vi "Derivative of intensity graph V1.0.vi"() -> ()   [LabVIEW 2016]
uses:
  <vilib>/Utility/miscctls.llb/LVOffsetAndMultiplierTypeDef.ctl
  <vilib>/Analysis/NI_AALPro.lvlib
panel:
  in  "Cursor.Visible ? 2":bool
  in  "Cursor.Visible ?":bool
  in  "Tab Control":T1(tab)=enum."Index linecut curve"
  out "All derivatives":cluster{dbl[], dbl[]}[](graph)
  out "All Data":cluster{dbl[], dbl[]}[](graph)
  out "Linecut of Data":dbl[](graph)=[-5.165548349618656e-08, -5.159647504832888e-08, -5.1548035526661304e-08, -5.148192440940621e-08, -5.1383318345099665e-08, -5.1286353274798515e-08, -5.1218371208053366e-08, -5.116268641366293e-08, -5.109130548013824e-08, -5.098742924360193e-08, -5.085517949337487e-08, -5.074484750756666e-08, -5.068211876052946e-08, -5.0617670460310636e-08, -5.052406640959861e-08, -5.0408820269667306e-08, -5.0295145102842986e-08, -5.022248512748516e-08, -5.0180627286568036e-08, -5.0122652084791704e-08, -5.0040971452737534e-08, -4.995074993072835e-08, -4.985441092029686e-08, -4.9765018529941685e-08, -4.9675366699941365e-08, -4.9564350089994913e-08, -4.947029200628265e-08, -4.941443648162086e-08, -4.9353383054520915e-08, -4.926843157132916e-08, -4.9167242647363985e-08, -4.9065280874750254e-08, -4.899516497811031e-08, -4.8946122255576085e-08, -4.8863182385243175e-08, -4.87432636505986e-08, -4.862626638254201e-08, -4.853802567987668e-08, -4.848543315041591e-08, -4.8426769491768916e-08, -4.8331422602193806e-08, -4.823856670019399e-08, -4.816860860479887e-08, -4.8102166770697064e-08, -4.802987848539934e-08, -4.793796883789405e-08, -4.781875406953681e-08, -4.771223992954938e-08, -4.763483877438248e-08, -4.754388789459166e-08, -4.7432043547268955e-08, -4.731969281618781e-08, -4.722403394999117e-08, -4.7168647720075765e-08, -4.7134074086052784e-08, -4.707674724162832e-08, -4.699229851817311e-08, -4.689341985858352e-08, -4.6792670550280276e-08, -4.670473526864287e-08, -4.661186261528778e-08, -4.6503181017626753e-08, -4.641773033998275e-08, -4.636383873714532e-08, -4.6302239747671046e-08, -4.6219178803954826e-08, -4.611830349088384e-08, -4.6008475468028e-08, -4.591595258925939e-08, -4.584258830545454e-08, -4.57565406467377e-08, -4.565177461639157e-08, -4.55465010012447e-08, -4.544778298049394e-08, -4.537022560498973e-08, -4.5294561734900574e-08, -4.51842662663245e-08, -4.50710244054238e-08, -4.498678438032247e-08, -4.4916903048519334e-08, -4.483955437949311e-08, -4.474237791949989e-08, -4.464581168364172e-08, -4.4578839630322026e-08, -4.453545408463023e-08, -4.449345444981521e-08, -4.4445241282709766e-08, -4.4385705029112496e-08, -4.432274008638454e-08, -4.428047295002768e-08, -4.4231581361464624e-08, -4.413781408332821e-08, -4.402319403819412e-08, -4.392601686965633e-08, -4.385863063612994e-08, -4.3801470329639925e-08, -4.371464154197799e-08, -4.3585122865865986e-08, -4.3460048915201843e-08, -4.337618346856069e-08, -4.331416381624075e-08, -4.3252734547339044e-08, -4.3178842629403106e-08, -4.309602498723277e-08, -4.302060377664933e-08, -4.2945197911975524e-08, -4.2853584205840277e-08, -4.274446242764889e-08, -4.2631638334099326e-08, -4.253330374780791e-08, -4.2464012166724194e-08, -4.240684288478342e-08, -4.2325780772523794e-08, -4.222915038694011e-08, -4.2144893670544885e-08, -4.207001139198109e-08, -4.197951570204532e-08, -4.186293064936822e-08, -4.175155954277796e-08, -4.167633885796429e-08, -4.161761529242304e-08, -4.154372126835706e-08, -4.145120843461285e-08, -4.134665858173513e-08, -4.1249818939228537e-08, -4.11753684692289e-08, -4.1091024655823804e-08, -4.0975882847820176e-08, -4.085292266614936e-08, -4.0742754209786083e-08, -4.0659009748824605e-08, -4.0591286871812844e-08, -4.050720526388395e-08, -4.040783116052655e-08, -4.032631292398029e-08, -4.026575037929934e-08, -4.020033236599087e-08, -4.0118832371796704e-08, -4.0017884803601105e-08, -3.992062274168703e-08, -3.985915456501376e-08, -3.980910502914425e-08, -3.973949905215017e-08, -3.965749923353381e-08, -3.9573475035086906e-08, -3.949800011829344e-08, -3.942955342618568e-08, -3.933789965676449e-08, -3.922077992498132e-08, -3.912218722513151e-08, -3.905296257274388e-08, -3.8992130231414786e-08, -3.892327433845437e-08, -3.882445359006842e-08, -3.871234332414376e-08, -3.861881128126975e-08, -3.853639914523126e-08, -3.8456071626752795e-08, -3.837040236955144e-08, -3.827509069359456e-08, -3.820089270678577e-08, -3.815510009217847e-08, -3.8094101565054805e-08, -3.8009604245617294e-08, -3.791565039339955e-08, -3.781772114946437e-08, -3.7735527934768004e-08, -3.764922395007989e-08, -3.752862986218264e-08, -3.739858140578617e-08, -3.729352807309609e-08, -3.722253575841222e-08, -3.717238799522547e-08, -3.710583846146186e-08, -3.6999146668920645e-08, -3.6896083204113855e-08, -3.682999300151662e-08, -3.6769350479570105e-08, -3.669548253247852e-08, -3.660576874233244e-08, -3.6510217859818705e-08, -3.644074722814453e-08, -3.638687764944132e-08, -3.63104746678855e-08, -3.622213670971757e-08, -3.614929360125362e-08, -3.608616338943413e-08, -3.6024629858553956e-08, -3.594304806568941e-08, -3.5824548620609036e-08, -3.571563766462648e-08, -3.5646256883374475e-08, -3.558942283879134e-08, -3.5529346267070896e-08, -3.546135688902753e-08, -3.538546477475565e-08, -3.5322051576189394e-08, -3.5267963006398924e-08, -3.518638711023153e-08, -3.5077382944481216e-08, -3.496386175795827e-08, -3.485415433070339e-08, -3.4764224144210785e-08, -3.4679024766190425e-08, -3.4569988051248505e-08, -3.445874551980504e-08, -3.437124888411822e-08, -3.4303495045724726e-08, -3.4241346286418414e-08, -3.415948871180689e-08, -3.404952931528982e-08, -3.395058866948328e-08, -3.387865260122285e-08, -3.379725534723817e-08, -3.3704385993142976e-08, -3.3611839290837744e-08, -3.3515668636009095e-08, -3.344473917229437e-08, -3.3391339751836916e-08, -3.3305173758579915e-08, -3.319985030525287e-08, -3.311949351003222e-08, -3.305718996268877e-08, -3.299190902530916e-08, -3.29144757103662e-08, -3.281945470454397e-08, -3.2734986427922816e-08, -3.267696636548646e-08, -3.261974075041499e-08, -3.253445721133879e-08, -3.2405981533870483e-08, -3.226814349082853e-08, -3.216969703090513e-08, -3.210322902432682e-08, -3.2034629006142696e-08, -3.196009883122792e-08, -3.190026803540523e-08, -3.186337349867941e-08, -3.183599113260375e-08, -3.178096045409717e-08, -3.167867261642787e-08, -3.155730568256794e-08, -3.144426242929421e-08, -3.134959422836359e-08, -3.126876064771173e-08, -3.118366897239564e-08, -3.109381626446461e-08, -3.102917302092374e-08, -3.0995226421904973e-08, -3.095257095643533e-08, -3.087830071872433e-08, -3.077292081721096e-08, -3.0663717622016714e-08, -3.0586800674701934e-08, -3.0519909704341385e-08, -3.0428417060716443e-08, -3.031994915876719e-08, -3.021478359451866e-08, -3.012696058420965e-08, -3.005164622346892e-08, -2.99653646597268e-08, -2.98668895432762e-08, -2.9783009507890182e-08, -2.971327345593366e-08, -2.9638758475141435e-08, -2.955588599747759e-08, -2.946114270188039e-08, -2.9371640281182034e-08, -2.9303969115742402e-08, -2.9228801497056452e-08, -2.9123987631820767e-08, -2.9006876333603397e-08, -2.889923136094302e-08, -2.8816560698415582e-08, -2.8755997304679404e-08, -2.868170895711246e-08, -2.8578856589791276e-08, -2.8481290945567485e-08, -2.8404508937544794e-08, -2.8333305132237064e-08, -2.8251321719996546e-08, -2.814739759659086e-08, -2.804734616398572e-08, -2.7985450603452592e-08, -2.794437289599192e-08, -2.7880983143687256e-08, -2.778577975169189e-08, -2.7681281818291328e-08, -2.7601390761100666e-08, -2.756031474905914e-08, -2.7516809263284313e-08, -2.7445445010736174e-08, -2.736270737442078e-08, -2.727763117497891e-08, -2.7197946311589063e-08, -2.7120970747323493e-08, -2.702555948420715e-08, -2.6911600850550554e-08, -2.6816481307868774e-08, -2.6753150958716478e-08, -2.6693381712429233e-08, -2.660865438773106e-08, -2.6487032872792765e-08, -2.6365426120953676e-08, -2.627675831719376e-08, -2.6195161209717578e-08, -2.6099676084656567e-08, -2.5986396512281783e-08, -2.586723331071279e-08, -2.57835600655147e-08, -2.5738347234919e-08, -2.5679780414312992e-08, -2.559371639968789e-08, -2.5508309281632726e-08, -2.542956210418315e-08, -2.536115018323055e-08, -2.529184664632403e-08, -2.5195566825791836e-08, -2.5098662406207293e-08, -2.502554277389618e-08, -2.495268948619173e-08, -2.486601204395687e-08, -2.4760906463117536e-08, -2.464420797588273e-08, -2.455796873847971e-08, -2.4512213051135366e-08, -2.446195521773658e-08, -2.439636233437496e-08, -2.433152093401889e-08, -2.4266100296247668e-08, -2.4206929169608104e-08, -2.4136895052437086e-08, -2.4023778821815217e-08, -2.389002406014159e-08, -2.3774983953668427e-08, -2.368055336512477e-08, -2.3594935263044867e-08, -2.3503552165209706e-08, -2.3400009391694284e-08, -2.3319671183307225e-08, -2.326801413303854e-08, -2.3193851922599745e-08, -2.3089762124699337e-08, -2.2977748645147562e-08, -2.287448718729575e-08, -2.2805841155513513e-08, -2.275507350669239e-08, -2.267630666531651e-08, -2.2570712541859644e-08, -2.246884853943456e-08, -2.238319963142675e-08, -2.2312650014034985e-08, -2.2236937256527653e-08, -2.2136623645915668e-08, -2.203940093476987e-08, -2.1966393859608153e-08, -2.1896426138264626e-08, -2.18147422517242e-08, -2.1713288461790726e-08, -2.159774261507225e-08, -2.1505223158569168e-08, -2.1440090810716427e-08, -2.135722698071537e-08, -2.1250197110569697e-08, -2.1149508545896832e-08, -2.1069737284153304e-08, -2.1021898347111185e-08, -2.0981827622678454e-08, -2.0906481810483677e-08, -2.081466042512085e-08, -2.0744894567369e-08, -2.0697507729396806e-08, -2.0649843890112284e-08, -2.05641959407945e-08, -2.0432780646470743e-08, -2.0313373023767253e-08, -2.02326793255826e-08, -2.0150153361860347e-08, -2.0050066917813527e-08, -1.9938173404966368e-08, -1.9826619698408437e-08, -1.9741389771251036e-08, -1.967331644749085e-08, -1.95967010561806e-08, -1.9509851465096232e-08, -1.9424175649438275e-08, -1.9349724040100852e-08, -1.928195903350066e-08, -1.9198926357104354e-08, -1.909415070580926e-08, -1.900076819853445e-08, -1.8935772355636684e-08, -1.887772440051576e-08, -1.880849990199008e-08, -1.8716035876576055e-08, -1.8615119560084032e-08, -1.8539278487844478e-08, -1.8483419365321094e-08, -1.8415566535526765e-08, -1.832510175957605e-08, -1.8229381708746358e-08, -1.815210665530519e-08, -1.809714875140782e-08, -1.8025438038450318e-08, -1.7912436087299903e-08, -1.778786376701964e-08, -1.7676558631855445e-08, -1.758833435530881e-08, -1.751481606287522e-08, -1.7430530511459936e-08, -1.734447890831483e-08, -1.728565292959516e-08, -1.724369041238253e-08, -1.7186846008023987e-08, -1.710887230229723e-08, -1.7012745268222465e-08, -1.6921762346041743e-08, -1.686304001386004e-08, -1.6808203193226277e-08, -1.672867349459447e-08, -1.6640778286783097e-08, -1.6562465665146048e-08, -1.649307278281337e-08, -1.6414833641115934e-08, -1.6309502048004952e-08, -1.61925964935726e-08, -1.609988846453436e-08, -1.6034955655819488e-08, -1.597788376143784e-08, -1.5911344518422905e-08, -1.5815056064921685e-08, -1.5707127938219644e-08, -1.562759118775518e-08, -1.5567338292123593e-08, -1.549541054181991e-08, -1.539904415352674e-08, -1.5287688781456924e-08, -1.5197776224619042e-08, -1.5146163077683e-08, -1.5095507250291076e-08, -1.5021699555668288e-08, -1.4936991122444403e-08, -1.4846799461274123e-08, -1.4760015182297042e-08, -1.4678721453769657e-08, -1.4587630679287875e-08, -1.4492109148486224e-08, -1.4409655145686607e-08, -1.4332472274496851e-08, -1.4241520844757481e-08, -1.4137195331797136e-08, -1.4032510557306588e-08, -1.3954690342415332e-08, -1.3919879069510388e-08, -1.3889309773205139e-08, -1.3823012457910934e-08, -1.3714343763670049e-08, -1.3582616877477166e-08, -1.3473385978376832e-08, -1.3386722465806217e-08, -1.3284322927542685e-08, -1.3174843825390438e-08, -1.3087360353305362e-08, -1.3017520458568193e-08, -1.2949180336720338e-08, -1.2863364089578688e-08, -1.2752478393040186e-08, -1.2658016472807758e-08, -1.2594156545535696e-08, -1.2520618128319783e-08, -1.2426862223755474e-08, -1.2317782313911042e-08, -1.220651974100887e-08, -1.2127053532708653e-08, -1.2064271764396918e-08, -1.196981883072222e-08, -1.1856468163056788e-08, -1.1761603413309386e-08, -1.1683132319558236e-08, -1.1621355819165963e-08, -1.156305707516347e-08, -1.14781929922653e-08, -1.1392304836951796e-08, -1.1329073021039129e-08, -1.1265580236056948e-08, -1.1187897553103228e-08, -1.1092851453069643e-08, -1.0990244049742042e-08, -1.0914928210011268e-08, -1.0872738616645667e-08, -1.0819224965385265e-08, -1.0739920005576415e-08, -1.0656878439927393e-08, -1.0582297862333001e-08, -1.0525987000314038e-08, -1.046173190721331e-08, -1.035651321823925e-08, -1.0238490401322905e-08, -1.0142799526292181e-08, -1.0067932025393349e-08, -1.0004321757125447e-08, -9.933526685958005e-09, -9.835479815980103e-09, -9.74113193796887e-09, -9.673965130826426e-09, -9.595856144937196e-09, -9.492685060150827e-09, -9.38001971308705e-09, -9.279626260057881e-09, -9.221005382762921e-09, -9.184733555278047e-09, -9.120500989160431e-09, -9.025840506429946e-09, -8.932145614276231e-09, -8.852814358161073e-09, -8.797257647216194e-09, -8.749182103393222e-09, -8.667510487589974e-09, -8.572131951998509e-09, -8.496003882705925e-09, -8.424339528976975e-09, -8.343028285603508e-09, -8.24444902268272e-09, -8.13673920615525e-09, -8.056210752229678e-09, -7.997060976058544e-09, -7.911666948356154e-09, -7.801761162441733e-09, -7.694240051854376e-09, -7.601870735996258e-09, -7.529865694439582e-09, -7.449058981336632e-09, -7.338705121025062e-09, -7.229611012815972e-09, -7.145876566963134e-09, -7.082864620891759e-09, -7.024614500089476e-09, -6.951867022733208e-09, -6.874594933851745e-09, -6.821708339567503e-09, -6.782236362020187e-09, -6.71496685057371e-09, -6.612975105890926e-09, -6.492186408345851e-09, -6.382466294769023e-09, -6.313830390278918e-09, -6.262288499418076e-09, -6.195925443521832e-09, -6.110803983354142e-09, -6.017022581261779e-09, -5.939045629598735e-09, -5.879541807848321e-09, -5.811558024582396e-09, -5.725505923244007e-09, -5.639454359574765e-09, -5.557365579869371e-09, -5.473226258843006e-09, -5.385698585309521e-09, -5.283104016875587e-09, -5.177306044841199e-09, -5.097556145014069e-09, -5.036758797957208e-09, -4.959833982811004e-09, -4.856620356001262e-09, -4.749323397412903e-09, -4.667162153152393e-09, -4.619967902875641e-09, -4.563515319858662e-09, -4.462281670697812e-09, -4.342261614056037e-09, -4.237722427729048e-09, -4.162116380117339e-09, -4.098193178167314e-09, -4.012628380297198e-09, -3.912399887414766e-09, -3.831032296848197e-09, -3.764491213194643e-09, -3.683048717285538e-09, -3.581587892597002e-09, -3.474758155371428e-09, -3.390621002711189e-09, -3.346544366975868e-09, -3.306975431276149e-09, -3.23612362083844e-09, -3.141011790352063e-09, -3.047715291345525e-09, -2.973666465440155e-09, -2.90106529832146e-09, -2.800406246753331e-09, -2.682960275309979e-09, -2.586555073968205e-09, -2.513061440493684e-09, -2.438404873476138e-09, -2.351155718865382e-09, -2.241614750612168e-09, -2.126484408342364e-09, -2.040778864849992e-09, -1.975659952098716e-09, -1.906832555145674e-09, -1.834123821516362e-09, -1.759463244262756e-09, -1.692609976976152e-09, -1.645098126506399e-09, -1.590227738036847e-09, -1.51023407784728e-09, -1.428122415161914e-09, -1.355893433074301e-09, -1.289712491412466e-09, -1.212518769511009e-09, -1.114195314563714e-09, -1.027258440256342e-09, -9.749573562469318e-10, -9.358149897646206e-10, -8.865887560862493e-10, -8.117209811156121e-10, -7.136088643152043e-10, -6.268052558608579e-10, -5.509458883830812e-10, -4.5272433744728223e-10, -3.4670744003115907e-10, -2.5562060907888193e-10, -1.802456561690418e-10, -1.3170070119795185e-10, -8.534646031427943e-11, -1.97221748159532e-12, 1.0702911783967736e-10, 2.074145219610546e-10, 2.7943939175116353e-10, 3.3284048931347274e-10, 4.0542859174716504e-10, 5.176666545079506e-10, 6.298976454006431e-10, 7.11220422290744e-10, 7.805686358108225e-10, 8.461792336775194e-10, 9.14387160859313e-10, 9.900564202975778e-10, 1.050569087455051e-09, 1.103004630149216e-09, 1.182610694953509e-09, 1.280592594562181e-09, 1.368126705827701e-09, 1.444887492044754e-09, 1.512039069376415e-09, 1.585737876032312e-09, 1.690752991508098e-09, 1.790048611808742e-09, 1.849358489923578e-09, 1.893431651587018e-09, 1.944764726401677e-09, 2.016152675107883e-09, 2.108019126485136e-09, 2.189088752967968e-09, 2.249821979029339e-09, 2.3219329664673e-09, 2.414508903205599e-09, 2.518258549812626e-09, 2.622091311361718e-09, 2.702563799344889e-09, 2.772830365595461e-09, 2.862581335270108e-09, 2.9576143499494e-09, 3.037685468324933e-09, 3.105862063168961e-09, 3.168069186313731e-09, 3.242946819642778e-09, 3.345965839430557e-09, 3.441113826887668e-09, 3.502845163517442e-09, 3.560724170002592e-09, 3.631853306784242e-09, 3.719571116542628e-09, 3.811352050396102e-09, 3.876886286800509e-09, 3.929268682573394e-09, 4.003104770069814e-09, 4.091938970397758e-09, 4.168538554649564e-09, 4.227957208515581e-09, 4.283240103261025e-09, 4.359254178364449e-09, 4.463785865416529e-09, 4.567479030693155e-09, 4.658969313917753e-09, 4.745262305191378e-09, 4.82937446468876e-09, 4.929871582345169e-09, 5.043455077590558e-09, 5.134895741920077e-09, 5.205542739940588e-09, 5.289058477878094e-09, 5.386858437935474e-09, 5.482805771909853e-09, 5.55949315015377e-09, 5.608523481805763e-09, 5.671057092445083e-09, 5.769958292267436e-09, 5.871197734370865e-09, 5.953511081499268e-09, 6.015922494623362e-09, 6.077181521628707e-09, 6.171390758149761e-09, 6.294392061441708e-09, 6.402879921346237e-09, 6.480325477609046e-09, 6.549126724375836e-09, 6.624447468468814e-09, 6.711557477120861e-09, 6.794422700616358e-09, 6.853227742245409e-09, 6.912520892289393e-09, 6.996232652067696e-09, 7.095250013434509e-09, 7.18520347002369e-09, 7.245433904663959e-09, 7.288980296799043e-09, 7.354137200806825e-09, 7.45303678945682e-09, 7.556287447751107e-09, 7.643818196631916e-09, 7.715781020436906e-09, 7.78780589050345e-09, 7.888972496478919e-09, 7.99695053605507e-09, 8.072769681841774e-09, 8.134823951704828e-09, 8.210898347367893e-09, 8.301254424185938e-09, 8.389622965628687e-09, 8.455749446628741e-09, 8.502022973956721e-09, 8.560622189762535e-09, 8.64599930006857e-09, 8.744848059800704e-09, 8.844448875332305e-09, 8.92464394910288e-09, 8.991216485501273e-09, 9.081119093518476e-09, 9.19292961268178e-09, 9.29428865813295e-09, 9.374403964092157e-09, 9.444952857702575e-09, 9.520971977856758e-09, 9.615463210536748e-09, 9.714054523333864e-09, 9.786293254846991e-09, 9.841912693162742e-09, 9.896566843421918e-09, 9.947149924592754e-09, 9.994616264799956e-09, 1.0038338114463675e-08, 1.0094584610428635e-08, 1.0189037829990057e-08, 1.0312403734907897e-08, 1.0424863001982345e-08, 1.0510740471611777e-08, 1.0585912383990889e-08, 1.0677004578914405e-08, 1.080164064793784e-08, 1.0920797945838383e-08, 1.1000374040290892e-08, 1.1063741414466672e-08, 1.1127280243413212e-08, 1.1203122363644999e-08, 1.1294119497114395e-08, 1.1367538061859904e-08, 1.1420972210913038e-08, 1.1501051917307735e-08, 1.1616009539291896e-08, 1.1730468693596893e-08, 1.1819617281948062e-08, 1.1869222197180777e-08, 1.1913664125702742e-08, 1.2005190537066129e-08, 1.212134930589453e-08, 1.2217230630482162e-08, 1.2292640289393664e-08, 1.2364464758756383e-08, 1.2451938910811e-08, 1.2561812702431805e-08, 1.2657618607528987e-08, 1.2722981037915e-08, 1.2794872104465586e-08, 1.2878909459264943e-08, 1.29643128760194e-08, 1.305367616540603e-08, 1.31317888148128e-08, 1.3214504595448504e-08, 1.3329630442937902e-08, 1.344925847086242e-08, 1.3538428697299023e-08, 1.3597615519818674e-08, 1.3642301278170928e-08, 1.3701804191457527e-08, 1.379644107163972e-08, 1.3888495004408155e-08, 1.3950722205668911e-08, 1.4016185759978389e-08, 1.4099167582052692e-08, 1.419594778249263e-08, 1.4293174973164673e-08, 1.4360888059867663e-08, 1.4410175084427285e-08, 1.4473458161670337e-08, 1.4553428126254261e-08, 1.4640526798762081e-08, 1.4726882553011164e-08, 1.4796032727714565e-08, 1.486406910834282e-08, 1.4962238518432254e-08, 1.5070776726736442e-08, 1.5170990591558302e-08, 1.5264351702306638e-08, 1.534498861629775e-08, 1.5427915765550982e-08, 1.5526093889452664e-08, 1.5610561457256137e-08, 1.566609500654794e-08, 1.5724712774777637e-08, 1.580219450012296e-08, 1.5895100930536846e-08, 1.598781240433693e-08, 1.6049363117497512e-08, 1.610205298722932e-08, 1.6181909025158218e-08, 1.627159114496131e-08, 1.6345892903623263e-08, 1.640107643911102e-08, 1.6453516160546824e-08, 1.653421436527301e-08, 1.6649838058751213e-08, 1.6758592216232775e-08, 1.6836043746249e-08, 1.6907558133365794e-08, 1.6994527914833242e-08, 1.7102605496307657e-08, 1.7209115690165052e-08, 1.728748617832701e-08, 1.7368427869322018e-08, 1.7479556870475946e-08, 1.7600282116838245e-08, 1.7701135643215318e-08, 1.776479366625892e-08, 1.779965272620044e-08, 1.7840223212940547e-08, 1.7903628262606855e-08, 1.7970292181195662e-08, 1.8033676873356743e-08, 1.8101084435164234e-08, 1.8179237058837476e-08, 1.828044511901662e-08, 1.83860681374998e-08, 1.846161959334024e-08, 1.8509743919255925e-08, 1.8558697700881797e-08, 1.8624485968386326e-08, 1.8708365959710625e-08, 1.8790775065715824e-08, 1.885508374541348e-08, 1.8935038650383928e-08, 1.9046203753822493e-08, 1.9157078943833073e-08, 1.9251401617539353e-08, 1.9323034156881114e-08, 1.9385889316442635e-08, 1.9477429827888835e-08, 1.959888339309868e-08, 1.9708038884969772e-08, 1.978449613231618e-08, 1.985201294855826e-08, 1.9936292539619277e-08, 2.0045087866665358e-08, 2.0156936404943194e-08, 2.0242924032773942e-08, 2.0312949555024964e-08, 2.0387440310560902e-08, 2.0473770139021454e-08, 2.0568508225281878e-08, 2.0652699598592896e-08, 2.072336150384025e-08, 2.080714048805633e-08, 2.0910518014698132e-08, 2.0998072021995798e-08, 2.105011101567836e-08, 2.1088451133660523e-08, 2.114789834989974e-08, 2.1242719823543973e-08, 2.1342343946097603e-08, 2.1415709478654806e-08, 2.1477606819268027e-08, 2.155217525294655e-08, 2.1642896415492614e-08, 2.174084798594475e-08, 2.1825526403649565e-08, 2.1887872460836682e-08, 2.195509883348865e-08, 2.2041680259582098e-08, 2.2127428908633932e-08, 2.2200911096072432e-08, 2.226152409341246e-08, 2.232753261251945e-08, 2.2426145512634688e-08, 2.25477122633337e-08, 2.26521768272383e-08, 2.2721464767246816e-08, 2.2781706475209588e-08, 2.285974025258537e-08, 2.295695562902798e-08, 2.3040454697963323e-08, 2.3096410277596145e-08, 2.3166304241596258e-08, 2.3258966818466787e-08, 2.3355847753265965e-08, 2.3447579120961695e-08, 2.3516782007237627e-08, 2.3570059599775604e-08, 2.3633754222398075e-08, 2.3715853007581443e-08, 2.3811254335935492e-08, 2.3914059513583777e-08, 2.400618692262407e-08, 2.408864151016274e-08, 2.418819220112119e-08, 2.4286540487748527e-08, 2.4358275552841362e-08, 2.4426401038544805e-08, 2.4509072683106424e-08, 2.4608785976614754e-08, 2.4714172577996937e-08, 2.4797082849690735e-08, 2.4861363466135757e-08, 2.4939445612417945e-08, 2.503052903500613e-08, 2.51209153488853e-08, 2.5208710681047462e-08, 2.5275695241613537e-08, 2.533628835239673e-08, 2.5420423445030705e-08, 2.5509140231936764e-08, 2.5585543565343013e-08, 2.5652624806960306e-08, 2.5721127015016193e-08, 2.58193542604177e-08, 2.5948280970236214e-08, 2.60557735425621e-08, 2.6116533293709993e-08, 2.6175701073850748e-08, 2.6265379266949066e-08, 2.637159847267614e-08, 2.6464275443934576e-08, 2.6520144970790018e-08, 2.657301158865007e-08, 2.6665662658819513e-08, 2.6776437850057243e-08, 2.6876991980407546e-08, 2.6959405480845765e-08, 2.7015958778167645e-08, 2.707461293095013e-08, 2.716561849051297e-08, 2.725104330937161e-08, 2.7302373818445058e-08, 2.7351933617211823e-08, 2.7424649746261914e-08, 2.752293661764218e-08, 2.762968998868858e-08, 2.7714649565560406e-08, 2.7783664392144016e-08, 2.786718262854518e-08, 2.7963237113274027e-08, 2.8061549412253194e-08, 2.816234677003543e-08, 2.8253698509290308e-08, 2.8347080597871444e-08, 2.845822718158825e-08, 2.8555541080819768e-08, 2.8620792124854756e-08, 2.8675201220653845e-08, 2.8734694032677198e-08, 2.881859870985676e-08, 2.892861225245981e-08, 2.901135352387524e-08, 2.9049513458021253e-08, 2.9099780669959583e-08, 2.9188379711238254e-08, 2.9300078378859404e-08, 2.940924112065755e-08, 2.9491812296930837e-08, 2.9569429250979316e-08, 2.9665310287048227e-08, 2.9766661403841886e-08, 2.986331781367818e-08, 2.994194982429144e-08, 3.000272564522448e-08, 3.007703586587533e-08, 3.0175350073138e-08, 3.0264432986166206e-08, 3.032641890684148e-08, 3.03860563464009e-08, 3.0460704974534834e-08, 3.0558814247851624e-08, 3.0666493121301305e-08, 3.074622028283432e-08, 3.081109753256946e-08, 3.0894500428730636e-08, 3.099622511830374e-08, 3.1100322170854616e-08, 3.118607118236865e-08, 3.1250276286423874e-08, 3.132384539970563e-08, 3.142291023593888e-08, 3.151585884444522e-08, 3.15903956832351e-08, 3.166126979811683e-08, 3.1738577569947074e-08, 3.183980471909239e-08, 3.195647841161593e-08, 3.205399777956031e-08, 3.2129229897358834e-08, 3.220854133174332e-08, 3.2299636752838934e-08, 3.239579752995867e-08, 3.248515310394872e-08, 3.2554220022136973e-08, 3.262373279513822e-08, 3.271076344149195e-08, 3.27981923019228e-08, 3.287726196384082e-08, 3.2947401134495176e-08, 3.301421650739765e-08, 3.309562993100744e-08, 3.3192335328059614e-08, 3.3281535877269185e-08, 3.3356430843238566e-08, 3.3437614858934866e-08, 3.353983264889862e-08, 3.3653120549134804e-08, 3.373881508549966e-08, 3.37773841545038e-08, 3.380545068722117e-08, 3.38582135832789e-08, 3.3939750512428064e-08, 3.402831675614398e-08, 3.409252471132529e-08, 3.414160955091702e-08, 3.421733527749169e-08, 3.432501774917496e-08, 3.443050499834897e-08, 3.451846683854177e-08, 3.4595523531649366e-08, 3.4686752551914756e-08, 3.481279491661033e-08, 3.49360523393685e-08, 3.501998856357453e-08, 3.508692665984605e-08, 3.516412627776246e-08, 3.5249823659431125e-08, 3.5338671110880154e-08, 3.542246816371117e-08, 3.5498779137415576e-08, 3.55894001749335e-08, 3.568890828911401e-08, 3.57751655640434e-08, 3.5844229875154074e-08, 3.589100749877654e-08, 3.595040051632697e-08, 3.6058771542569716e-08, 3.6177795520554056e-08, 3.626811650757857e-08, 3.633724677216587e-08, 3.640001265069852e-08, 3.647886693178206e-08, 3.6585984382430124e-08, 3.667693437670797e-08, 3.672535437231855e-08, 3.677047007768697e-08, 3.6830007572563136e-08, 3.69093382117945e-08, 3.701088217158553e-08, 3.710262041591134e-08, 3.718763013733632e-08, 3.7288729858617413e-08, 3.7388728402058916e-08, 3.7471265111082846e-08, 3.754663082388097e-08, 3.762663462482375e-08, 3.772083113834913e-08, 3.783171262902289e-08, 3.792546938039102e-08, 3.7985638879833045e-08, 3.80406414543943e-08, 3.8104830145835404e-08, 3.818988388133581e-08, 3.82902514388834e-08, 3.8370914577858356e-08, 3.8439752610406954e-08, 3.853412386617366e-08, 3.86485492476408e-08, 3.8756004625228107e-08, 3.88521418807705e-08, 3.8936115738334386e-08, 3.9024241118458894e-08, 3.9133976145567996e-08, 3.923774612432202e-08, 3.9313800703537645e-08, 3.937264190052518e-08, 3.943450174618713e-08, 3.951966375033713e-08, 3.962510237381826e-08, 3.971505791038223e-08, 3.977897178842526e-08, 3.985381546409646e-08, 3.995136136142911e-08, 4.005658027500406e-08, 4.014548277955852e-08, 4.019349690705462e-08, 4.023769069368033e-08, 4.032754314433714e-08, 4.0446296583144695e-08, 4.0555878957906824e-08, 4.0638833786187884e-08, 4.069725662620517e-08, 4.0762681071245344e-08, 4.085713765987981e-08, 4.094254878223259e-08, 4.099552228917106e-08, 4.10458022884179e-08, 4.111207729905143e-08, 4.120423052626266e-08, 4.130684195325961e-08, 4.13775778777784e-08, 4.143167007324635e-08, 4.151689598552298e-08, 4.1627012737623015e-08, 4.172891310720141e-08, 4.181081040158764e-08, 4.1875270611546905e-08, 4.194449124282775e-08, 4.203305784739945e-08, 4.21188600563364e-08, 4.21892381692549e-08, 4.22491609728867e-08, 4.2312737667997236e-08, 4.2404113480995726e-08, 4.251392405837233e-08, 4.260745587915246e-08, 4.268557238471463e-08, 4.277709296592051e-08, 4.2883482690344295e-08, 4.2989211147298195e-08, 4.30755220942012e-08, 4.313521420562231e-08, 4.320879035307412e-08, 4.3319268360154966e-08, 4.3441330103612357e-08, 4.3549485288525866e-08, 4.3622348555642996e-08, 4.3665007325065834e-08, 4.372123302929115e-08, 4.3812166217420045e-08, 4.389905750396691e-08, 4.395723700856061e-08, 4.400805030268893e-08, 4.407570377058768e-08, 4.4178309558806875e-08, 4.4286844550471064e-08, 4.4359629299087154e-08, 4.4414387225044866e-08, 4.4482986856557294e-08, 4.457653980460206e-08, 4.468755362177491e-08, 4.479451797524183e-08, 4.4884509376667604e-08, 4.4977369984743175e-08, 4.50962569342116e-08, 4.5219161914033986e-08, 4.531279456484088e-08, 4.5372620448601086e-08, 4.5429824386888904e-08, 4.551728108846942e-08, 4.5610189027528465e-08, 4.5670641205839105e-08, 4.570736009124178e-08, 4.5753178788246316e-08, 4.5834694392456525e-08, 4.594025397053122e-08, 4.6025546651073455e-08, 4.608356611197761e-08, 4.615586693935353e-08, 4.625575587601021e-08, 4.6361097996096765e-08, 4.645410730174644e-08, 4.65138592005244e-08, 4.6552335931444475e-08, 4.6617439332131655e-08, 4.6715236431143914e-08, 4.681447731141728e-08, 4.690320740704745e-08, 4.6984426361638847e-08, 4.706645307284108e-08, 4.716158808692999e-08, 4.724573359633799e-08, 4.7298379061707716e-08, 4.735694378157567e-08, 4.744600831959383e-08, 4.755438152663565e-08, 4.766164269352361e-08, 4.774478631784626e-08, 4.781217707615645e-08, 4.7898943345741315e-08, 4.800908813466092e-08, 4.8112768638607634e-08, 4.81935803463964e-08, 4.8252695592614195e-08, 4.8320431848215856e-08, 4.842677441081415e-08, 4.853727676668916e-08, 4.8611390633610313e-08, 4.866265347419583e-08, 4.872109621965567e-08, 4.880816364182065e-08, 4.892095416901144e-08, 4.902307162807421e-08, 4.910895114367844e-08, 4.921541261837963e-08, 4.93363614876348e-08, 4.944136810564916e-08, 4.9522808341914866e-08, 4.9575158854426204e-08, 4.962338444352588e-08, 4.96731566993443e-08]
  in  "Y index for line cut curve":dbl=4.0
  out "Y value":string="Temp (K)= 700.0m"
  out "Linecut of derivative":cluster{dbl[], dbl[]}(graph)
  in  "Name":T2={"X"="Vsd (V)", "Y"="Temp (K)", "Z"="I (A)", "dZ/dX"="dI/dV (S)"}
  in  "Enum":T3(ring)=enum."dz/dx vs x"
  out "Derivative of Data":dbl[][](graph)
  out "Column number":i32=1230
  out "Row number":i32=18
  in  "Ex":T4={"Offset"=-0.00486, "Multiplier"=8e-06}
  in  "Ey":T4={"Offset"=0.9, "Multiplier"=-0.05}
  in  "Data":dbl[][](graph)=array1230x18[22140 elements]
  in  "Step for derivative":dbl=15.0
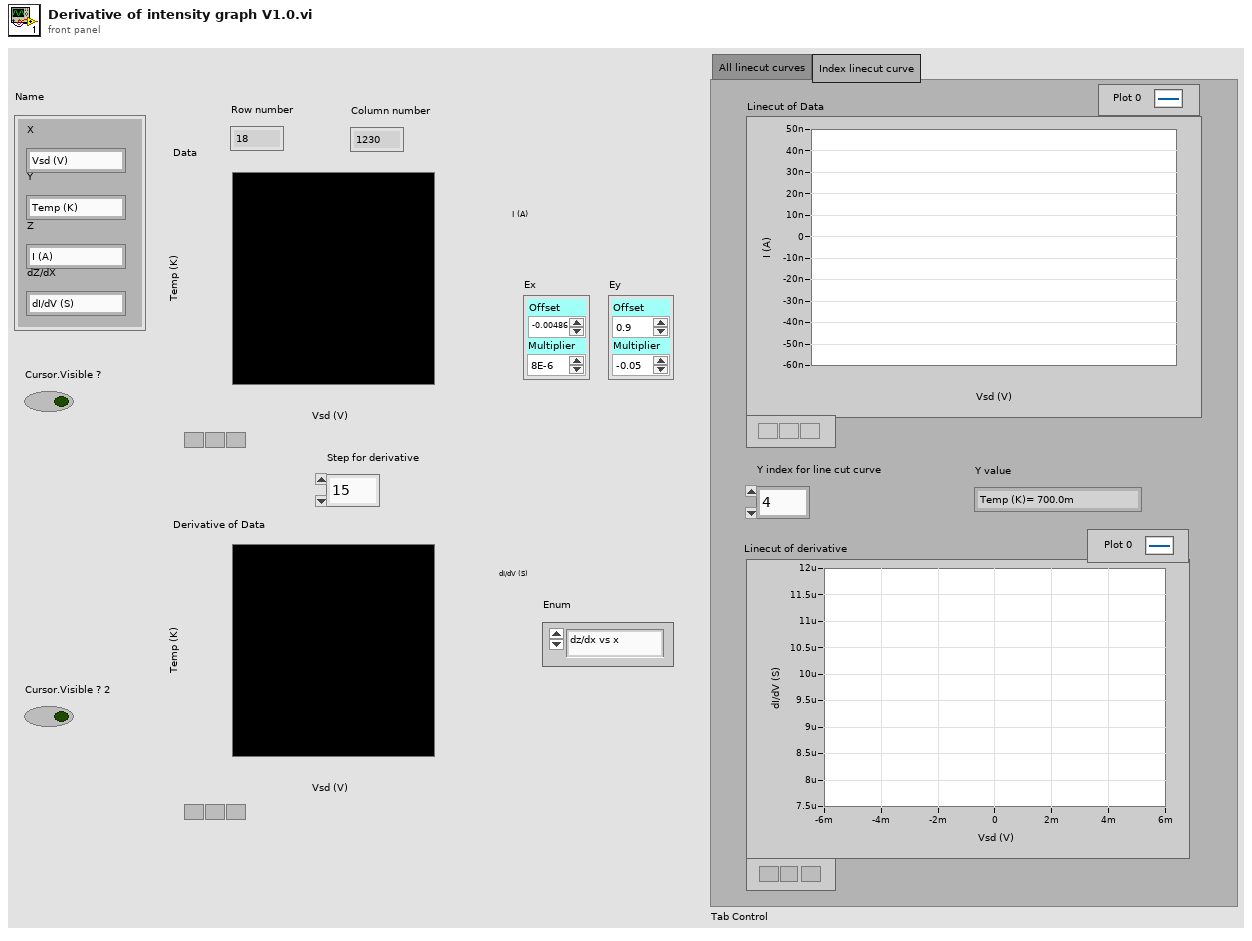
[diagram p1: front panel]
types:
  T1 = enum32{"All linecut curves", "Index linecut curve"}
  T2 = cluster{"X":string, "Y":string, "Z":string, "dZ/dX":string}
  T3 = enum16{"dz/dx vs z", "dz/dx vs x", "dx/dz vs z", "dx/dz vs x"}
  T4 = typedef "LVOffsetAndMultiplierTypeDef.ctl" = cluster{"Offset":dbl, "Multiplier":dbl}
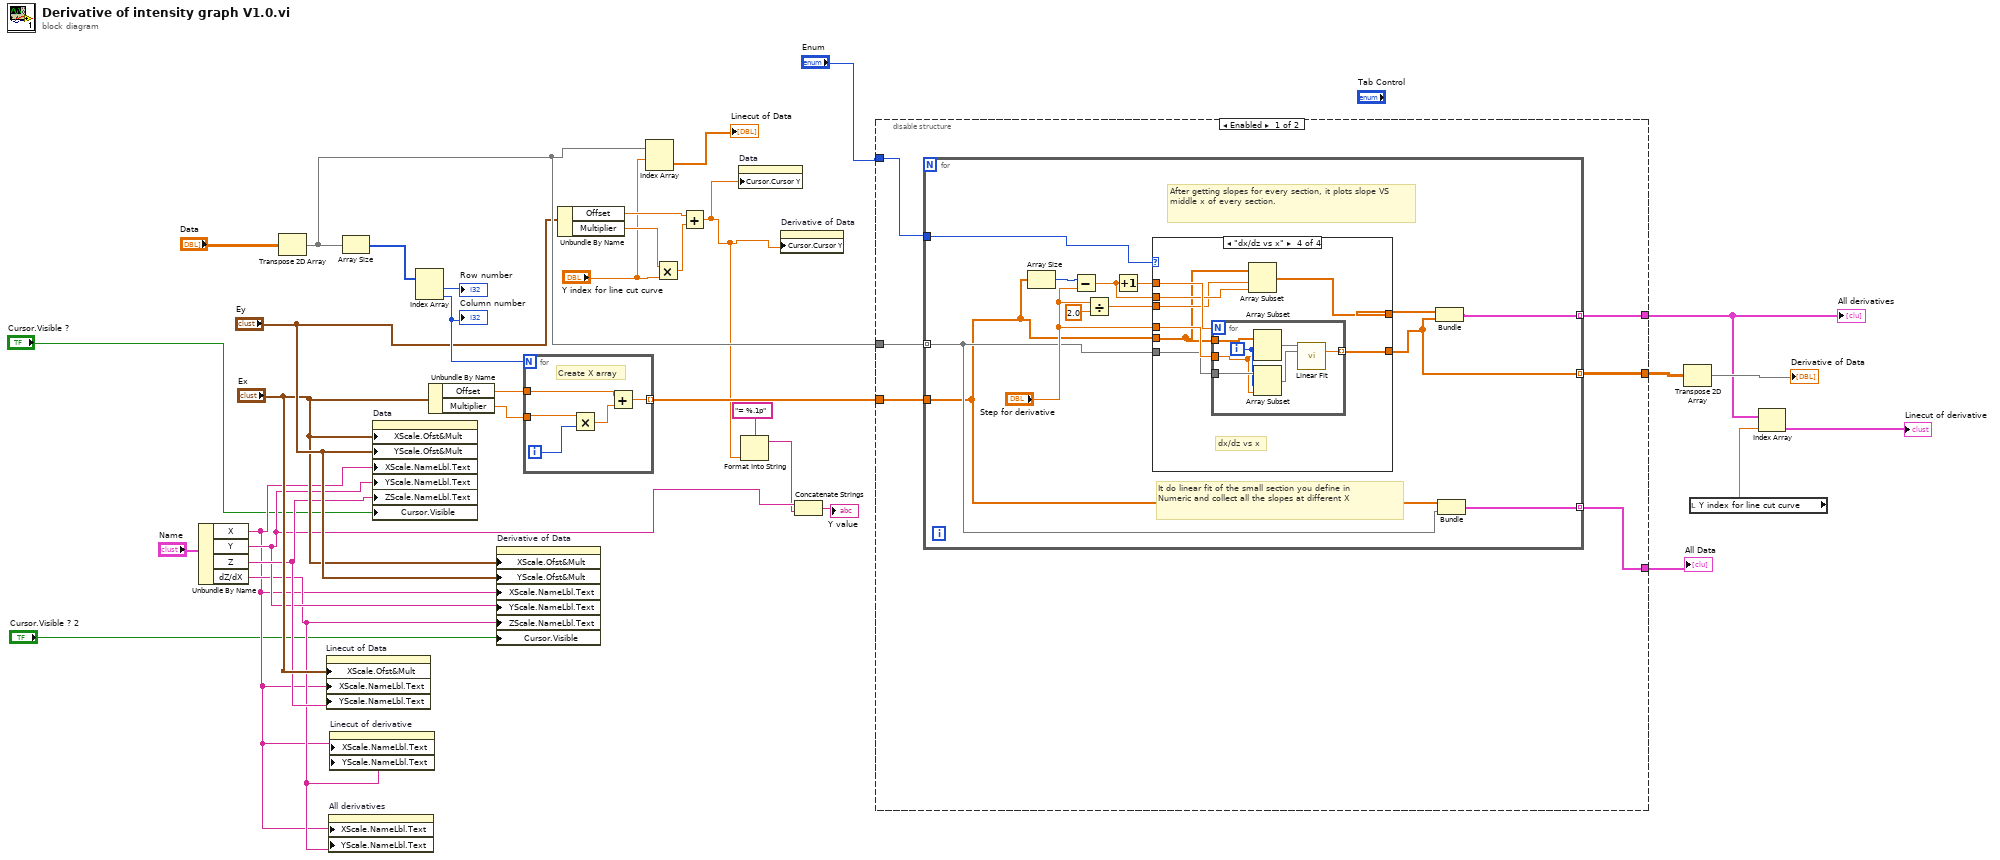
[diagram p0: block diagram]
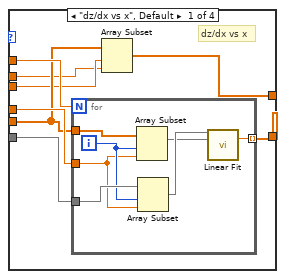
[diagram p2: hidden frame]
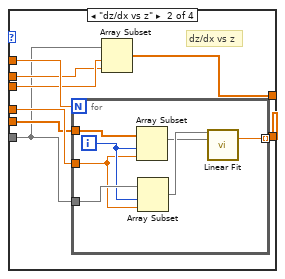
[diagram p3: hidden frame]
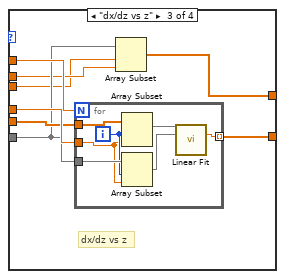
[diagram p4: hidden frame]
diagram:
  n1 = Unbundle By Name("Name") -> ("X"=w3:string, "Y"=w12:string, "Z"=w14:string, "dZ/dX"=w4:string)
  n2 = Transpose 2D Array(2D array="Data") -> (transposed array=w25:dbl[][])
  n3 = property on="Linecut of Data" class="WFGraph (strict)"("XScale.Ofst&Mult"="Ex", "XScale.NameLbl.Text"=w3, "YScale.NameLbl.Text"=w14) -> ()  [unwired: 2 in, 2 out]
  n4 = property on="All derivatives" class="XYGraph (strict)"("XScale.NameLbl.Text"=w3, "YScale.NameLbl.Text"=w4) -> ()  [unwired: 2 in, 2 out]
  n5 = property on="Linecut of derivative" class="XYGraph (strict)"("XScale.NameLbl.Text"=w3, "YScale.NameLbl.Text"=w4) -> ()  [unwired: 2 in, 2 out]
  n6 = Array Size(array=w25) -> (size(s)=w31:i32[])
  n7 = property on="Data" class="IntGraph (strict)"("XScale.Ofst&Mult"="Ex", "YScale.Ofst&Mult"="Ey", "XScale.NameLbl.Text"=w3, "YScale.NameLbl.Text"=w12, "ZScale.NameLbl.Text"=w14, "Cursor.Visible"="Cursor.Visible ?") -> ()  [unwired: 2 in, 2 out]
  n8 = Index Array(array=w31) -> (element #1=→"Row number":i32, element #2=w29:i32)  [unwired: 2 in]
  "Column number" <- w29
  n9 = Unbundle By Name("Ex") -> ("Offset"=w27:dbl, "Multiplier"=w28:dbl)
  n10 = property on="Derivative of Data" class="IntGraph (strict)"("XScale.Ofst&Mult"="Ex", "YScale.Ofst&Mult"="Ey", "XScale.NameLbl.Text"=w3, "YScale.NameLbl.Text"=w12, "ZScale.NameLbl.Text"=w4, "Cursor.Visible"="Cursor.Visible ? 2") -> ()  [unwired: 2 in, 2 out]
  n11 = for {
    N: w29 -> [_]
    tunnel: w28 -> [w38]
    tunnel: w27 -> [w36]
    tunnel: [w34] -> w26 mode=indexing
    i -> [w37]
    # "Create X array"
    n12 = Multiply(x=w38, y=w37) -> (x*y=w35:dbl)
    n13 = Add(x=w36, y=w35) -> (x+y=w34:dbl)
  }
  n14 = Unbundle By Name("Ey") -> ("Offset"=w22:dbl, "Multiplier"=w21:dbl)
  n15 = Index Array(array=w25, index (row)="Y index for line cut curve") -> (element=→"Linecut of Data":dbl[])  [unwired: 1 in]
  n16 = Multiply(x=w21, y="Y index for line cut curve") -> (x*y=w20:dbl)
  n17 = Add(x=w22, y=w20) -> (x+y=w10:dbl)
  n18 = property on="Data" class="IntGraph (strict)"("Cursor.Cursor Y"=w10) -> ()  [unwired: 2 in, 2 out]
  n19 = Format Into String(format string="= %.1p", w10) -> (resulting string=w8:string)  [unwired: 2 in, 1 out]
  n20 = property on="Derivative of Data" class="IntGraph (strict)"("Cursor.Cursor Y"=w10) -> ()  [unwired: 2 in, 2 out]
  n21 = Concatenate Strings(w12, w8) -> (→"Y value":string)
  n22 = disable-structure shown="Enabled" {
    disable-tunnel: "Enum" -> [w44 _]
    disable-tunnel: w26 -> [w43 _]
    disable-tunnel: w25 -> [w42 _]
    disable-tunnel: [w41 _] -> w16
    disable-tunnel: [w40 _] -> w7
    disable-tunnel: [w39 _] -> w13
    frame Enabled {
      n23 = for {
        tunnel: [w51] -> w40 mode=indexing
        tunnel: w44 -> [w50]
        tunnel: w43 -> [w46]
        tunnel: w42 -> [w47] mode=indexing
        tunnel: [w48] -> w41 mode=indexing
        tunnel: [w45] -> w39 mode=indexing
        # "After getting slopes for every section, it plots slope VS middle x of every section."
        # "It do linear fit of the small section you define in Numeric and collect all the slopes at different X"
        n24 = Array Size(array=w46) -> (size(s)=w49:i32)
        n25 = Subtract(x=w49, y="Step for derivative") -> (x-y=w53:dbl)
        n26 = Divide(x="Step for derivative", y=2.0) -> (x/y=w54:dbl)
        n27 = Increment(x=w53) -> (x+1=w57:dbl)
        n28 = case shown="\"dx/dz vs x\"" w50 {
          tunnel: w57 -> [w65 w80 w95 w110]
          tunnel: "Step for derivative" -> [w64 w79 w94 w109]
          tunnel: [w58 w74 w88 w104] -> w48
          tunnel: w46 -> [w62 w78 w93 w103]
          tunnel: w47 -> [w63 w73 w92 w108]
          tunnel: w54 -> [w61 w77 w90 w106]
          tunnel: w53 -> [w60 w76 w91 w107]
          tunnel: [w59 w75 w89 w105] -> w52
          frame "dz/dx vs x", Default {
            # "dz/dx vs x"
            n29 = for {
              N: w65 -> [_]
              tunnel: w62 -> [w72]
              tunnel: w63 -> [w71]
              tunnel: w64 -> [w69]
              tunnel: [w68] -> w58 mode=indexing
              i -> [w70]
              n30 = Array Subset(array=w72, index=w70, length=w69) -> (w66:dbl[])
              n31 = Array Subset(array=w71, index=w70, length=w69) -> (w67:dbl[])
              n32 = call <vilib>:"Linear Fit.vi"("Y"=w67, "X"=w66) -> ("slope"=w68:dbl)  [unwired: 9 in, 4 out]
            }
            n33 = Array Subset(array=w62, index=w61, length=w60) -> (w59:dbl[])
          }
          frame "dz/dx vs z" {
            # "dz/dx vs z"
            n34 = for {
              N: w80 -> [_]
              tunnel: w78 -> [w87]
              tunnel: w73 -> [w86]
              tunnel: w79 -> [w84]
              tunnel: [w83] -> w74 mode=indexing
              i -> [w85]
              n35 = Array Subset(array=w87, index=w85, length=w84) -> (w81:dbl[])
              n36 = Array Subset(array=w86, index=w85, length=w84) -> (w82:dbl[])
              n37 = call <vilib>:"Linear Fit.vi"("Y"=w82, "X"=w81) -> ("slope"=w83:dbl)  [unwired: 9 in, 4 out]
            }
            n38 = Array Subset(array=w73, index=w77, length=w76) -> (w75:dbl[])
          }
          frame "dx/dz vs z" {
            # "dx/dz vs z"
            n39 = for {
              N: w95 -> [_]
              tunnel: w93 -> [w102]
              tunnel: w92 -> [w101]
              tunnel: w94 -> [w99]
              tunnel: [w98] -> w88 mode=indexing
              i -> [w100]
              n40 = Array Subset(array=w102, index=w100, length=w99) -> (w97:dbl[])
              n41 = Array Subset(array=w101, index=w100, length=w99) -> (w96:dbl[])
              n42 = call <vilib>:"Linear Fit.vi"("Y"=w97, "X"=w96) -> ("slope"=w98:dbl)  [unwired: 9 in, 4 out]
            }
            n43 = Array Subset(array=w92, index=w90, length=w91) -> (w89:dbl[])
          }
          frame "dx/dz vs x" {
            # "dx/dz vs x"
            n44 = for {
              N: w110 -> [_]
              tunnel: w103 -> [w117]
              tunnel: w108 -> [w116]
              tunnel: w109 -> [w114]
              tunnel: [w113] -> w104 mode=indexing
              i -> [w115]
              n45 = Array Subset(array=w117, index=w115, length=w114) -> (w112:dbl[])
              n46 = Array Subset(array=w116, index=w115, length=w114) -> (w111:dbl[])
              n47 = call <vilib>:"Linear Fit.vi"("Y"=w112, "X"=w111) -> ("slope"=w113:dbl)  [unwired: 9 in, 4 out]
            }
            n48 = Array Subset(array=w103, index=w106, length=w107) -> (w105:dbl[])
          }
        }
        n49 = Bundle(w52, w48) -> (w51:cluster{dbl[], dbl[]})  [unwired: 1 in]
        n50 = Bundle(w46, w47) -> (w45:cluster{dbl[], dbl[]})  [unwired: 1 in]
      }
    }
    frame Disabled {
    }
  }
  "All derivatives" <- w7
  "All Data" <- w13
  n51 = Transpose 2D Array(2D array=w16) -> (transposed array=→"Derivative of Data":dbl[][])
  n52 = local read "Y index for line cut curve"() -> (w5:dbl)
  n53 = Index Array(array=w7, index=w5) -> (element=→"Linecut of derivative":cluster{dbl[], dbl[]})
